vi "run method.vi"(8 "error in (no error)":errorcluster, 10 "JSON Value in":variant, 11 "Method Manager in":refnum<class "Method Loader.lvclass">) -> (0 "error out":errorcluster, 2 "JSON Value out":variant, 3 "Method Manager out":refnum<class "Method Loader.lvclass">)   [LabVIEW 2020, in "JSON-RPC Lib.lvlib" / "Method Loader.lvclass"]
uses:
  Method Loader.lvclass
  Method Loader.lvclass/Method Loader.ctl
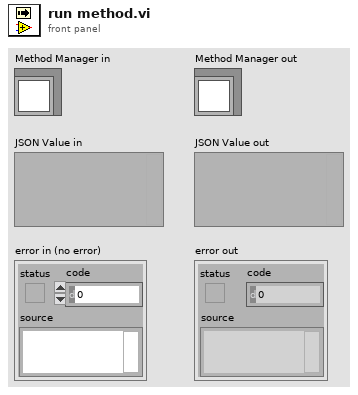
[diagram p1: front panel]
types:
  T1 = typedef "JSON-RPC Lib.lvlib/Method Loader.lvclass/method type.ctl" = refnum<vi>
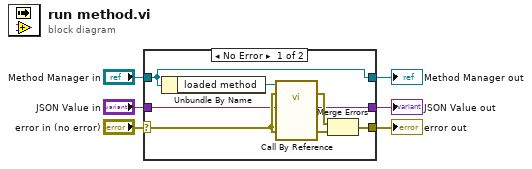
[diagram p0: block diagram]
diagram:
  n1 = case shown="No Error" "error in (no error)" {
    selector: "error in (no error)" -> [w12 w16]
    tunnel: [w11 w16] -> w5
    tunnel: [w10 w15] -> w3
    tunnel: "Method Manager in" -> [w10 w15]
    tunnel: "JSON Value in" -> [w8 _]
    tunnel: [w7 _] -> w1
    frame No Error {
      n2 = Unbundle By Name(w10) -> ("loaded method"=w9:T1)
      n3 = call-by-ref "?"(reference=w9, error in=w12, 8:"error in (no error)"=w12, "params"=w8) -> (error out=w13:errorcluster, 0:"error out"=w14:errorcluster, "data"=w7:variant)  [unwired: 8 in, 1 out]
      n4 = Merge Errors(w13, w14) -> (w11:errorcluster)
    }
    frame Error {
    }
  }
  "error out" <- w5
  "Method Manager out" <- w3
  "JSON Value out" <- w1
